vi "correct_profile.vi"() -> ()   [LabVIEW 2010]
panel:
  out "iteration":i16
  out "number not converged":i16
  in  "results file":string
  in  "grid size for z*":i16=32
  in  "grid size for u* and v*":i16=40
  in  "orientation":enum16{"uv", "uw"}(ring)
  in  "input file":string
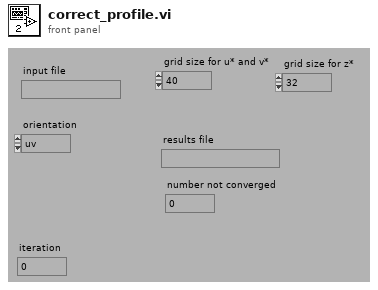
[diagram p1: front panel]
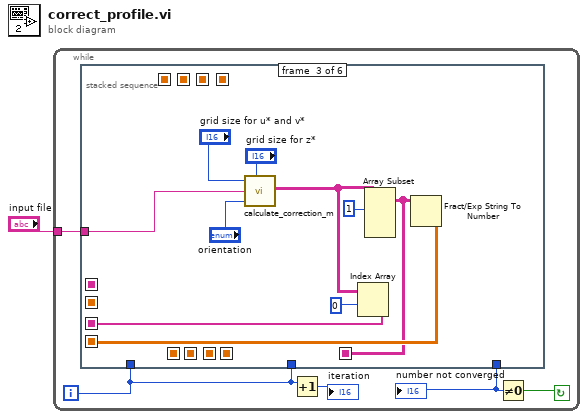
[diagram p0: block diagram]
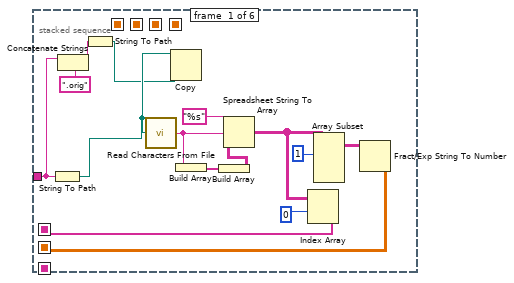
[diagram p2: hidden frame]
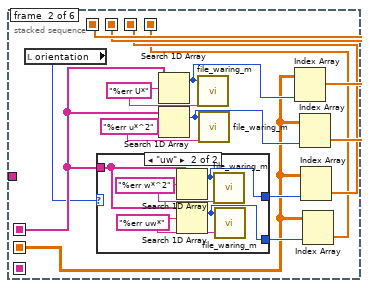
[diagram p3: hidden frame]
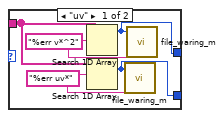
[diagram p4: hidden frame]
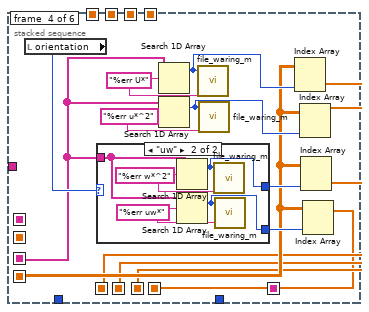
[diagram p5: hidden frame]
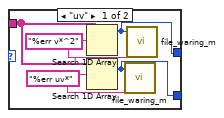
[diagram p6: hidden frame]
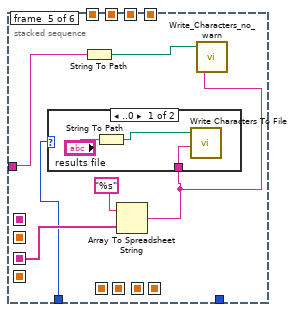
[diagram p7: hidden frame]
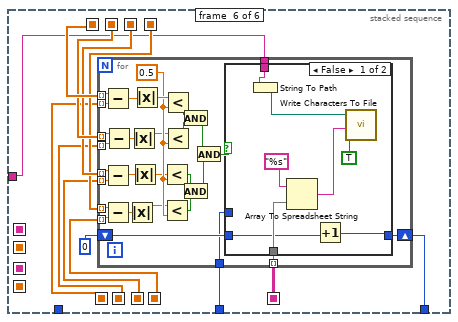
[diagram p9: hidden frame]
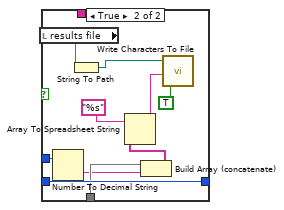
[diagram p10: hidden frame]
diagram:
  n1 = while {
    tunnel: "input file" -> [w6]
    i -> [w3]
    stop <- w5 continue-if-true
    n2 = stacked-sequence {
      seq-local: [w13 _ _ _ _ _] -> [_ w32 _ _ _ _]
      seq-local: [w12 _ _ _ _ _] -> [_ w26 _ _ _ _]
      seq-local: [_ _ w48 _ _ _] -> [_ _ _ w59 w82 _]
      seq-local: [_ _ w47 _ _ _] -> [_ _ _ w60 _ _]
      seq-local: [_ w25 _ _ _ _] -> [_ _ _ _ _ w99]
      seq-local: [_ w24 _ _ _ _] -> [_ _ _ _ _ w98]
      seq-local: [_ w23 _ _ _ _] -> [_ _ _ _ _ w97]
      seq-local: [_ w22 _ _ _ _] -> [_ _ _ _ _ w96]
      seq-local: [_ _ _ w58 _ _] -> [_ _ _ _ _ w95]
      seq-local: [_ _ _ w57 _ _] -> [_ _ _ _ _ w94]
      seq-local: [_ _ _ w56 _ _] -> [_ _ _ _ _ w93]
      seq-local: [_ _ _ w55 _ _] -> [_ _ _ _ _ w92]
      seq-local: [_ _ w46 _ _ _] -> [_ _ _ _ _ w90]
      tunnel: w6 -> [w11 _ w45 _ w80 w91]
      tunnel: [_ _ _ _ _ w88] -> w4
      tunnel: w3 -> [_ _ _ _ w79 _]
      tunnel: w3 -> [_ _ _ _ _ w87]
      frame #0 {
        n3 = String To Path(string=w11) -> (path=w8:path)
        n4 = Concatenate Strings(w11, ".orig") -> (w9:string)
        n5 = String To Path(string=w9) -> (path=w7:path)
        n6 = call <vilib>:"Read Characters From File.vi"("file path (dialog if empty)"=w8) -> ("character string"=w18:string)  [unwired: 5 in, 3 out]
        n7 = Copy(10:w7, 11:w8) -> ()  [unwired: 3 in, 3 out]
        n8 = Build Array(w18) -> (w21:string[])
        n9 = Build Array(w21) -> (w20:string[][])
        n10 = Spreadsheet String To Array(format string="%s", spreadsheet string=w18, array type (2D Dbl)=w20) -> (array=w14:string[][])  [unwired: 1 in]
        n11 = Index Array(array=w14, index (row)=0) -> (element=w13:string[])  [unwired: 1 in]
        n12 = Array Subset(array=w14, index (row)=1) -> (w15:string[][])  [unwired: 3 in]
        n13 = Fract/Exp String To Number(string=w15) -> (number=w12:dbl[][])  [unwired: 3 in, 1 out]
      }
      frame #1 {
        w33 = "%err u*^2"
        w34 = "%err U*"
        n14 = local read "orientation"() -> (w31:enum16{"uv", "uw"})
        n15 = case shown="\"uw\"" w31 {
          tunnel: w32 -> [w37 w42]
          tunnel: [w36 w41] -> w29
          tunnel: [w35 w40] -> w28
          frame "uv" {
            w39 = "%err uv*"
            w38 = "%err v*^2"
            n16 = Search 1D Array(1D array=w37, element=w38) -> (index of element=w36:i32)  [unwired: 1 in]
            n17 = Search 1D Array(1D array=w37, element=w39) -> (index of element=w35:i32)  [unwired: 1 in]
            n18 = call "file_waring_m.vi"("item not found"=w39, "index"=w35) -> ()  [unwired: 3 in]
            n19 = call "file_waring_m.vi"("item not found"=w38, "index"=w36) -> ()  [unwired: 3 in]
          }
          frame "uw" {
            w44 = "%err uw*"
            w43 = "%err w*^2"
            n20 = Search 1D Array(1D array=w42, element=w43) -> (index of element=w41:i32)  [unwired: 1 in]
            n21 = Search 1D Array(1D array=w42, element=w44) -> (index of element=w40:i32)  [unwired: 1 in]
            n22 = call "file_waring_m.vi"("item not found"=w43, "index"=w41) -> ()  [unwired: 3 in]
            n23 = call "file_waring_m.vi"("item not found"=w44, "index"=w40) -> ()  [unwired: 3 in]
          }
        }
        n24 = Search 1D Array(1D array=w32, element=w34) -> (index of element=w30:i32)  [unwired: 1 in]
        n25 = Search 1D Array(1D array=w32, element=w33) -> (index of element=w27:i32)  [unwired: 1 in]
        n26 = call "file_waring_m.vi"("item not found"=w34, "index"=w30) -> ()  [unwired: 3 in]
        n27 = call "file_waring_m.vi"("item not found"=w33, "index"=w27) -> ()  [unwired: 3 in]
        n28 = Index Array(array=w26, index (col)=w30) -> (element=w25:dbl[])  [unwired: 1 in]
        n29 = Index Array(array=w26, index (col)=w27) -> (element=w24:dbl[])  [unwired: 1 in]
        n30 = Index Array(array=w26, index (col)=w29) -> (element=w23:dbl[])  [unwired: 1 in]
        n31 = Index Array(array=w26, index (col)=w28) -> (element=w22:dbl[])  [unwired: 1 in]
      }
      frame #2 {
        n32 = call "calculate_correction_m.vi"("grid size for u* and v*"="grid size for u* and v*", "grid size for z*"="grid size for z*", "input file"=w45, "orientation"="orientation") -> ("Results"=w49:string[][])  [unwired: 3 in]
        n33 = Index Array(array=w49, index (row)=0) -> (element=w48:string[])  [unwired: 1 in]
        n34 = Array Subset(array=w49, index (row)=1) -> (w46:string[][])  [unwired: 3 in]
        n35 = Fract/Exp String To Number(string=w46) -> (number=w47:dbl[][])  [unwired: 3 in, 1 out]
      }
      frame #3 {
        w66 = "%err u*^2"
        w67 = "%err U*"
        n36 = local read "orientation"() -> (w65:enum16{"uv", "uw"})
        n37 = case shown="\"uw\"" w65 {
          tunnel: w59 -> [w70 w75]
          tunnel: [w69 w74] -> w63
          tunnel: [w68 w73] -> w62
          frame "uv" {
            w72 = "%err uv*"
            w71 = "%err v*^2"
            n38 = Search 1D Array(1D array=w70, element=w71) -> (index of element=w69:i32)  [unwired: 1 in]
            n39 = Search 1D Array(1D array=w70, element=w72) -> (index of element=w68:i32)  [unwired: 1 in]
            n40 = call "file_waring_m.vi"("item not found"=w72, "index"=w68) -> ()  [unwired: 3 in]
            n41 = call "file_waring_m.vi"("item not found"=w71, "index"=w69) -> ()  [unwired: 3 in]
          }
          frame "uw" {
            w77 = "%err uw*"
            w76 = "%err w*^2"
            n42 = Search 1D Array(1D array=w75, element=w76) -> (index of element=w74:i32)  [unwired: 1 in]
            n43 = Search 1D Array(1D array=w75, element=w77) -> (index of element=w73:i32)  [unwired: 1 in]
            n44 = call "file_waring_m.vi"("item not found"=w76, "index"=w74) -> ()  [unwired: 3 in]
            n45 = call "file_waring_m.vi"("item not found"=w77, "index"=w73) -> ()  [unwired: 3 in]
          }
        }
        n46 = Search 1D Array(1D array=w59, element=w67) -> (index of element=w64:i32)  [unwired: 1 in]
        n47 = Search 1D Array(1D array=w59, element=w66) -> (index of element=w61:i32)  [unwired: 1 in]
        n48 = call "file_waring_m.vi"("item not found"=w67, "index"=w64) -> ()  [unwired: 3 in]
        n49 = call "file_waring_m.vi"("item not found"=w66, "index"=w61) -> ()  [unwired: 3 in]
        n50 = Index Array(array=w60, index (col)=w64) -> (element=w58:dbl[])  [unwired: 1 in]
        n51 = Index Array(array=w60, index (col)=w61) -> (element=w57:dbl[])  [unwired: 1 in]
        n52 = Index Array(array=w60, index (col)=w63) -> (element=w56:dbl[])  [unwired: 1 in]
        n53 = Index Array(array=w60, index (col)=w62) -> (element=w55:dbl[])  [unwired: 1 in]
      }
      frame #4 {
        n54 = String To Path(string=w80) -> (path=w78:path)
        n55 = Array To Spreadsheet String(array=w82, 3:"%s") -> (spreadsheet string=w81:string)  [unwired: 1 in]
        n56 = case shown="..0" w79 {
          tunnel: w81 -> [w86 _]
          frame ..0 {
            n57 = String To Path(string="results file") -> (path=w84:path)
            n58 = call <vilib>:"Write Characters To File.vi"("character string"=w86, "file path (dialog if empty)"=w84) -> ()  [unwired: 3 in, 1 out]
          }
          frame 1.. {
          }
        }
        n59 = call "Write_Characters_no_warn.vi"("character string"=w81, "file path (dialog if empty)"=w78) -> ()  [unwired: 3 in, 1 out]
      }
      frame #5 {
        n60 = for {
          tunnel: w99 -> [w128] mode=indexing
          tunnel: w98 -> [w126] mode=indexing
          tunnel: w97 -> [w124] mode=indexing
          tunnel: w96 -> [w122] mode=indexing
          tunnel: w95 -> [w127] mode=indexing
          tunnel: w94 -> [w125] mode=indexing
          tunnel: w93 -> [w123] mode=indexing
          tunnel: w92 -> [w121] mode=indexing
          tunnel: w91 -> [w104]
          tunnel: w90 -> [w103] mode=indexing
          shift-right: [w101] -> w88
          shift-left: 0 -> [w102]
          tunnel: w87 -> [w100]
          w118 = 0.5
          n61 = Subtract(x=w128, y=w127) -> (x-y=w120:dbl)
          n62 = Subtract(x=w124, y=w123) -> (x-y=w108:dbl)
          n63 = Subtract(x=w122, y=w121) -> (x-y=w110:dbl)
          n64 = Subtract(x=w126, y=w125) -> (x-y=w106:dbl)
          n65 = Absolute Value(x=w110) -> (abs(x)=w111:dbl)
          n66 = Absolute Value(x=w106) -> (abs(x)=w107:dbl)
          n67 = Absolute Value(x=w108) -> (abs(x)=w109:dbl)
          n68 = Absolute Value(x=w120) -> (abs(x)=w119:dbl)
          n69 = Less?(x=w109, y=w118) -> (x < y?=w113:bool)
          n70 = Less?(x=w111, y=w118) -> (x < y?=w112:bool)
          n71 = Less?(x=w119, y=w118) -> (x < y?=w117:bool)
          n72 = Less?(x=w107, y=w118) -> (x < y?=w116:bool)
          n73 = And(x=w117, y=w116) -> (x .and. y?=w115:bool)
          n74 = And(x=w113, y=w112) -> (x .and. y?=w114:bool)
          n75 = And(x=w115, y=w114) -> (x .and. y?=w105:bool)
          n76 = case shown="False" w105 {
            tunnel: w104 -> [w131 _]
            tunnel: w103 -> [w134 w141]
            tunnel: w102 -> [w133 w143]
            tunnel: [w132 w143] -> w101
            tunnel: w100 -> [_ w140]
            frame False {
              n77 = String To Path(string=w131) -> (path=w129:path)
              n78 = Array To Spreadsheet String(array=w134, 3:"%s") -> (spreadsheet string=w135:string)  [unwired: 1 in]
              n79 = Increment(x=w133) -> (x+1=w132:i32)
              n80 = call <vilib>:"Write Characters To File.vi"("append to file? (new file:F)"=TRUE, "character string"=w135, "file path (dialog if empty)"=w129) -> ()  [unwired: 2 in, 1 out]
            }
            frame True {
              n81 = local read "results file"() -> (w142:string)
              n82 = Number To Decimal String(number=w140) -> (decimal integer string=w139:string)  [unwired: 1 in]
              n83 = String To Path(string=w142) -> (path=w137:path)
              n84 = Build Array (concatenate)(w141, w139) -> (w138:string[])
              n85 = Array To Spreadsheet String(array=w138, 3:"%s") -> (spreadsheet string=w145:string)  [unwired: 1 in]
              n86 = call <vilib>:"Write Characters To File.vi"("append to file? (new file:F)"=TRUE, "character string"=w145, "file path (dialog if empty)"=w137) -> ()  [unwired: 2 in, 1 out]
            }
          }
        }
      }
    }
    "number not converged" <- w4
    n87 = Increment(x=w3) -> (x+1=→"iteration":i32)
    n88 = Not Equal To 0?(x=w4) -> (x != 0?=w5:bool)
  }
